vi "GetCurrentWindowHandle.vi"(1 "window title":string) -> (0 "hWnd":u32)   [LabVIEW 2009]
doc: "Get current window's handle"
uses:
  User32.dll
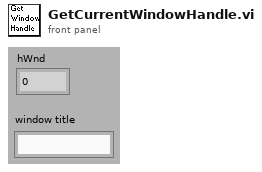
[diagram p1: front panel]
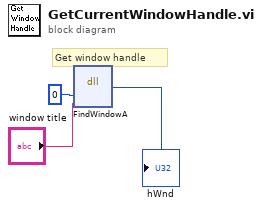
[diagram p0: block diagram]
diagram:
  # "Get window handle"
  n1 = dll-call lib="user32.dll" fn="FindWindowA"("lpszClassName"=0, "lpszWindowName"="window title") -> ("hWnd"=→"hWnd":u32)  [unwired: 5 in, 2 out]
